vi "打断循环方案.vi"() -> ()   [LabVIEW 2018]
panel:
  out "毫秒计时值":u32
  in  "继续执行":bool
  in  "停止循环":bool
  out "循环状态":bool
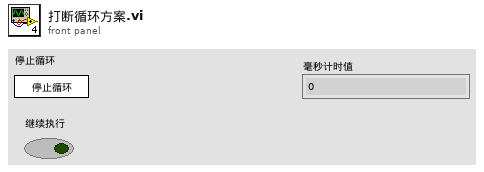
[diagram p1: front panel]
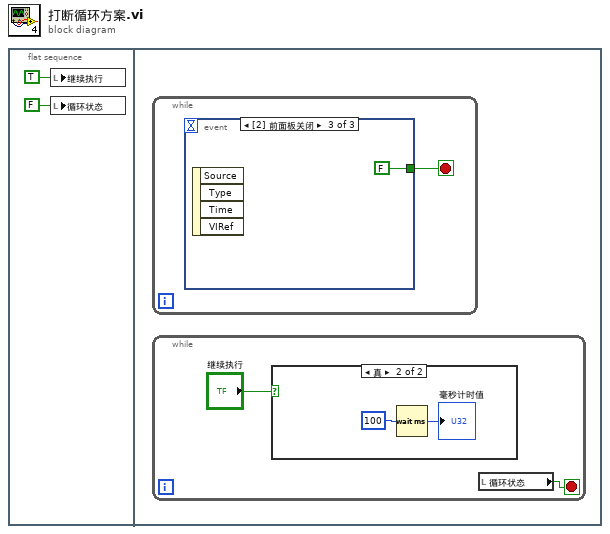
[diagram p0: block diagram]
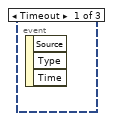
[diagram p3: hidden frame]
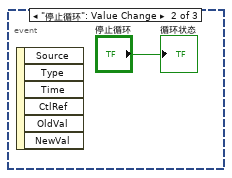
[diagram p4: hidden frame]
diagram:
  n1 = flat-sequence {
    frame #0 {
      n2 = local write "继续执行"(TRUE ("继续执行")) -> ()
      n3 = local write "循环状态"(FALSE ("循环状态")) -> ()
    }
    frame #1 {
      n4 = while {
        stop <- w7 stop-if-true
        n5 = event shown="[2] 前面板关闭" {
          selector: _ -> [_ _ _]
          dyn-events: _ -> [_ _ _]
          timeout: _ -> [_ _ _]
          tunnel: [_ _ FALSE] -> w7
          event Timeout {
            n6 = event-data() -> ()  [unwired: 1 in, 3 out]
          }
          event "停止循环": Value Change {
            n7 = event-data() -> ()  [unwired: 1 in, 6 out]
            "循环状态" <- "停止循环"
          }
          event Panel Close {
            n8 = event-data() -> ()  [unwired: 1 in, 4 out]
          }
        }
      }
      n9 = while {
        stop <- w4 stop-if-true
        n10 = case shown="真" "继续执行" {
          frame False {
          }
          frame True {
            n11 = Wait (ms)(milliseconds to wait=u32 100 ("等待时间（毫秒）")) -> (millisecond timer value=→"毫秒计时值":u32)
          }
        }
        n12 = local read "循环状态"() -> (w4:bool)
      }
    }
  }
